vi "Get Acquired Data16.vi"(8 "error in (no error)":errorcluster, 10 "size":u32, 11 "arr in":u16[](array[numeric])) -> (0 "error out":errorcluster, 2 "function return":u32, 3 "arr out":u16[](array[numeric]))   [LabVIEW 2014, in "atmcd32d.lvlib"]
uses:
  atmcd32d.lvlib
  atmcd32d.dll
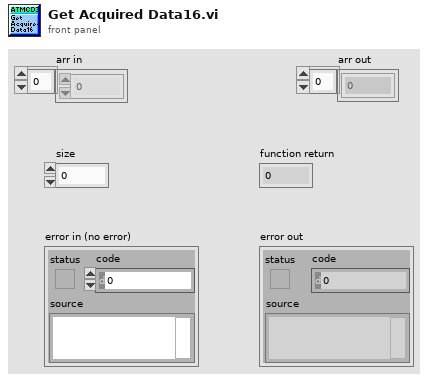
[diagram p1: front panel]
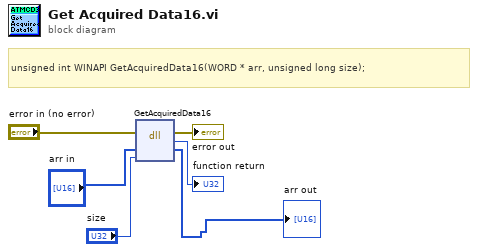
[diagram p0: block diagram]
diagram:
  # "unsigned int WINAPI GetAcquiredData16(WORD * arr, unsigned long size);"
  n1 = dll-call lib="C:/Users/Lambda2/Desktop/Testing/Lambda2-Testing/lib/Andorlib/atmcd32d.*" fn="GetAcquiredData16"(error in="error in (no error)", "arr"="arr in", "size"="size") -> (error out=→"error out":errorcluster, "return type"=→"function return":u32, "arr"=→"arr out":u16[])  [unwired: 3 in, 1 out]
